vi "Queue Decorate.vi"(10 "Queue Actor":refnum<class "Queue Actor.lvclass">, 11 "Hello World Queue in":refnum<class "Hello World Queue.lvclass">) -> (3 "Hello World Queue out":refnum<class "Hello World Queue.lvclass">)   [LabVIEW 2021, in "Hello World Queue.lvlib" / "Hello World Queue.lvclass"]
uses:
  Hello World Queue.lvclass
  Hello World Queue.lvclass/Hello World Queue.ctl
  Actor/Queue Actor/Queue Actor.lvclass
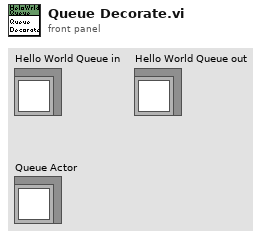
[diagram p1: front panel]
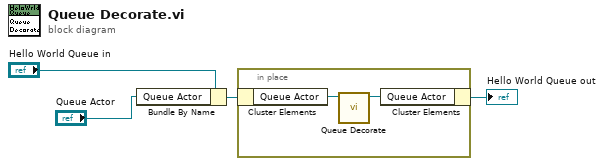
[diagram p0: block diagram]
diagram:
  n1 = Bundle By Name(cluster="Hello World Queue in", "Queue Actor"="Queue Actor") -> (w2:refnum<class "Hello World Queue.lvclass">)
  n2 = in-place {
    n3 = in-place-cluster #1(w2) -> ("Queue Actor"=w6:refnum<class "Queue Actor.lvclass">)
    n4 = call-dynamic "Queue Decorate.vi"("Queue Actor in"=w6) -> ("Queue Actor out"=w5:refnum<class "Queue Actor.lvclass">)  [unwired: 10 in]
    n5 = in-place-cluster #1("Queue Actor"=w5) -> (→"Hello World Queue out":refnum<class "Hello World Queue.lvclass">)
  }
